vi "Do.vi"(8 "error in (no error)":errorcluster, 10 "Actor in":refnum<class "Actor.lvclass">, 11 "Initialize request msg":refnum<class "Initialize request msg.lvclass">) -> (0 "error out":errorcluster, 2 "Actor out":refnum<class "Actor.lvclass">)   [LabVIEW 2015, in "Initialize request msg.lvclass"]
doc: "(<B>Filename</B>: Actor Framework.lvlib:Message.lvclass:Do.vi)\n\nDefines what a message does when it is received by an actor. Generally, a message instructs an actor to invoke one of its methods. By default, this method does nothing. A child class must override it to define behavior. Create a child class by using the Actor Framework Message Maker dialog box."
uses:
  Initialize request msg.lvclass
  <vilib>/ActorFramework/Actor/Actor.lvclass
  Gage digitizer actor.lvclass
  Initialize request msg.lvclass/Initialize request msg.ctl
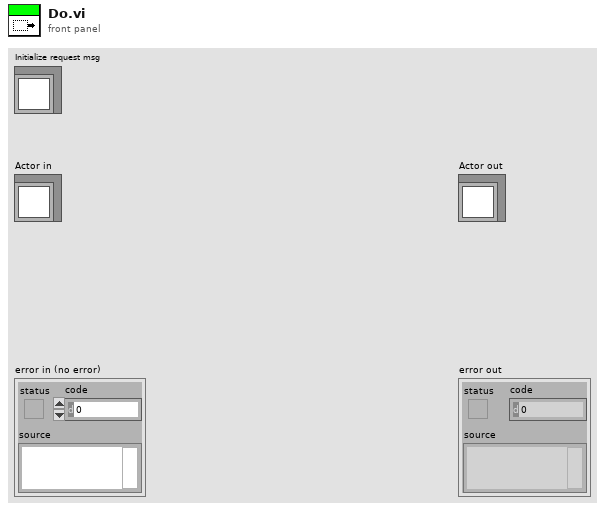
[diagram p1: front panel]
types:
  T1 = cluster{"Number of points":dbl, "Input Range":u32, "Trigger Level":i32, "Trigger source":bool}
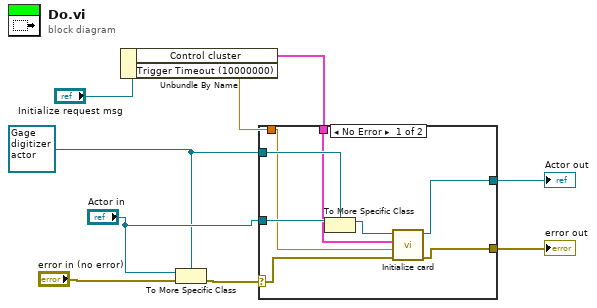
[diagram p0: block diagram]
diagram:
  w5 = refnum<class "Gage digitizer actor.lvclass"> refnum ("Gage digitizer actor in")
  n1 = Unbundle By Name("Initialize request msg") -> ("Control cluster"=w2:T1, "Trigger Timeout (10000000)"=w1:dbl)
  n2 = To More Specific Class(target class=w5, reference="Actor in", error in="error in (no error)") -> (error out=w8:errorcluster)  [unwired: 1 out]
  n3 = case shown="No Error" w8 {
    selector: w8 -> [w16 w19]
    tunnel: "Actor in" -> [w17 w18]
    tunnel: [w15 w19] -> w6
    tunnel: w5 -> [w14 _]
    tunnel: [w12 w18] -> w4
    tunnel: w2 -> [w11 _]
    tunnel: w1 -> [w10 _]
    frame No Error {
      n4 = To More Specific Class(target class=w14, reference=w17) -> (specific class reference=w13:refnum<class "Gage digitizer actor.lvclass">)  [unwired: 1 in, 1 out]
      n5 = call-dynamic "Initialize card.vi"("error in (no error)"=w16, "Trigger Timeout (10000000)"=w10, "Control cluster 2"=w11, "Gage digitizer actor in"=w13) -> ("error out"=w15:errorcluster, "Gage digitizer actor out"=w12:refnum<class "Gage digitizer actor.lvclass">)  [unwired: 6 in]
    }
    frame Error {
    }
  }
  "error out" <- w6
  "Actor out" <- w4
